vi "New.vi"(8 "error in (no error)":errorcluster, 9 "remote port or service name":u16=7776, 10 "address":string, 11 "LifterTCP in":refnum<class "LifterTCP.lvclass">) -> (0 "error out":errorcluster, 3 "LifterTCP out":refnum<class "LifterTCP.lvclass">)   [LabVIEW 2019, in "LifterTCP.lvclass"]
uses:
  LifterTCP.lvclass
  LifterTCP.lvclass/LifterTCP.ctl
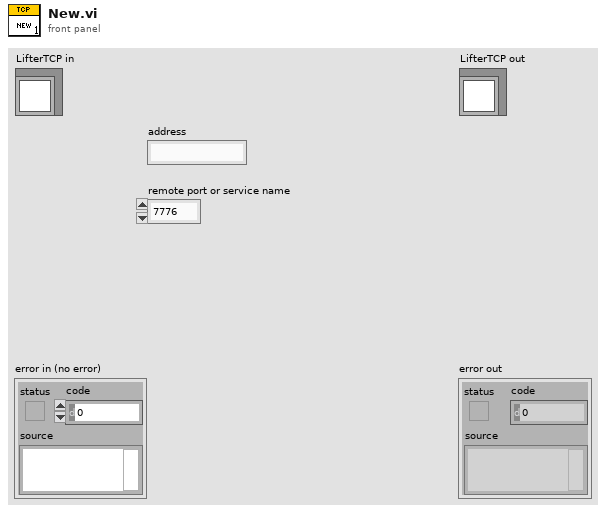
[diagram p1: front panel]
types:
  T1 = typedef "Semaphore RefNum" = refnum<k1>
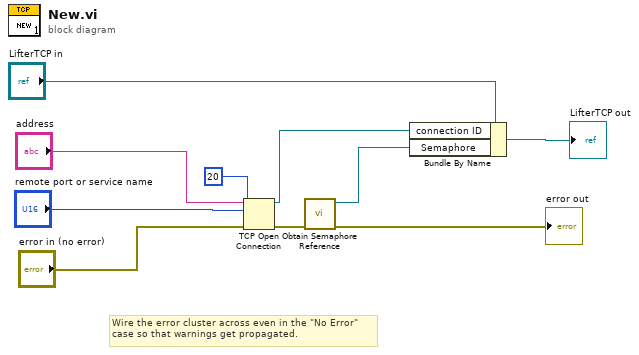
[diagram p0: block diagram]
diagram:
  # "Wire the error cluster across even in the \"No Error\"\ncase so that warnings get propagated."
  n1 = TCP Open Connection(address="address", remote port or service name="remote port or service name", timeout ms (60000)=20, error in (no error)="error in (no error)") -> (connection ID=w3:refnum<k5>, error out=w1:errorcluster)  [unwired: 1 in]
  n2 = call <vilib>:"Obtain Semaphore Reference.vi"("error in (no error)"=w1) -> ("error out"=→"error out":errorcluster, "semaphore"=w4:T1)  [unwired: 4 in, 1 out]
  n3 = Bundle By Name(cluster="LifterTCP in", "connection ID"=w3, "Semaphore"=w4) -> (→"LifterTCP out":refnum<class "LifterTCP.lvclass">)
